vi "Select Fiducial From Set.vi"(8 "error in":errorcluster, 9 "Selection Criteria":enum16{"Single", "Top", "Bottom"}(ring), 10 "Fiducial Centers":refnum<class "Vec3d Class.lvclass">[](array[class])) -> (0 "error out":errorcluster, 2 "Selected Fiducial":refnum<class "Vec3d Class.lvclass">)   [LabVIEW 2011]
uses:
  Vec3d Class/Vec3d Class.lvclass
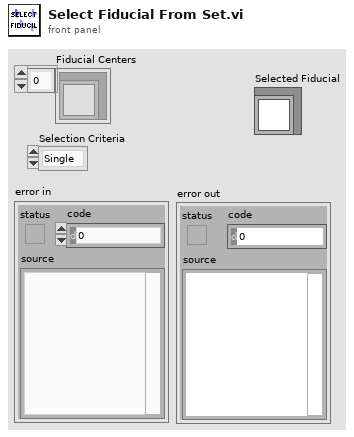
[diagram p1: front panel]
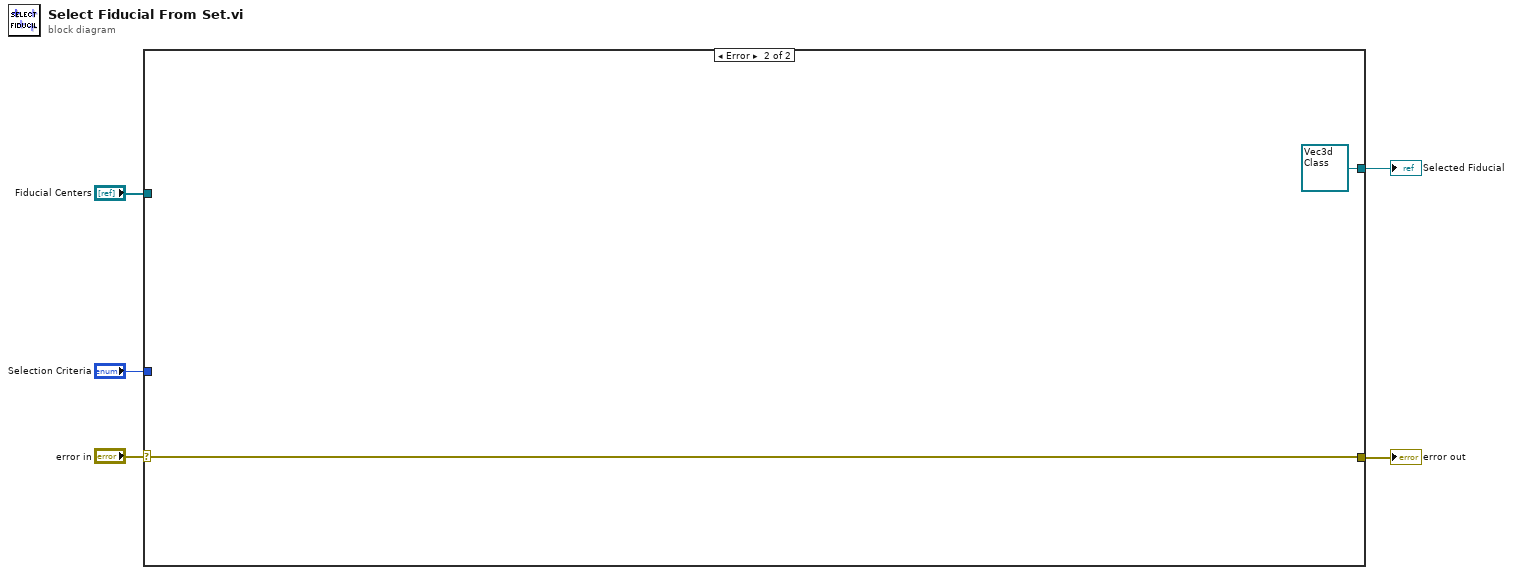
[diagram p0: block diagram]
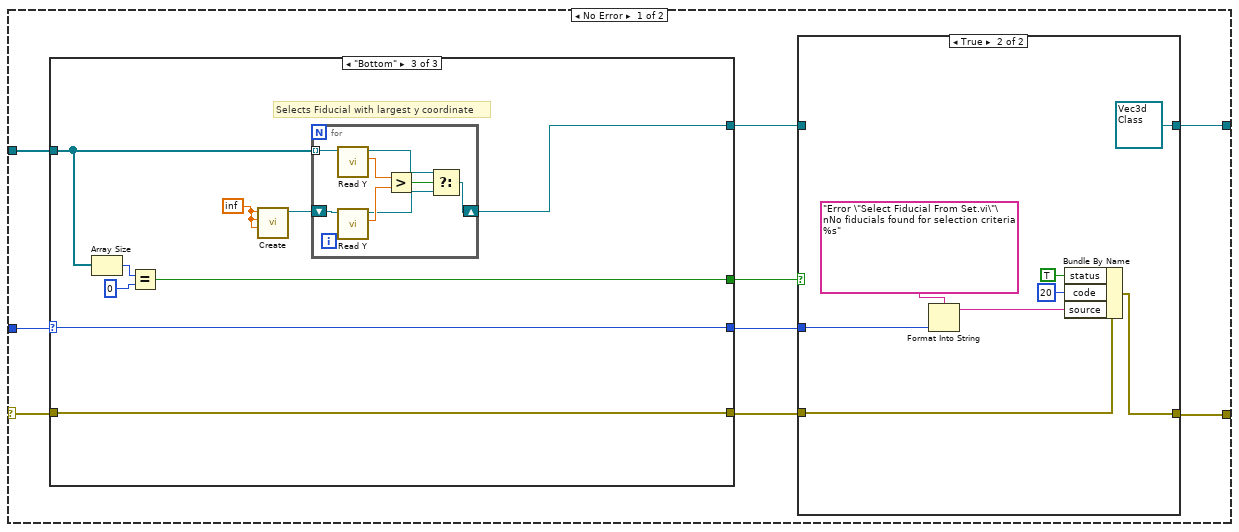
[diagram p2: hidden frame]
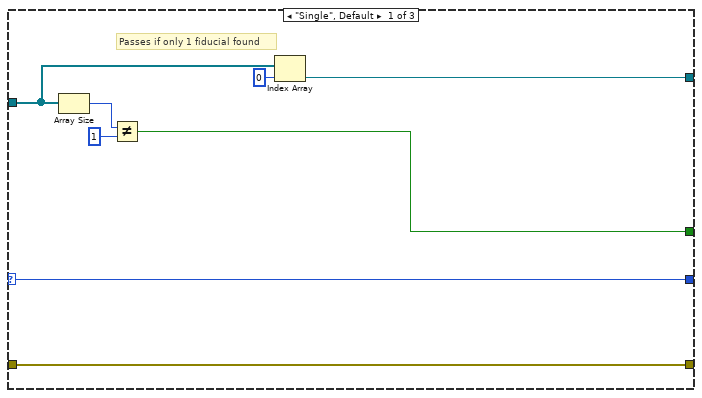
[diagram p3: hidden frame]
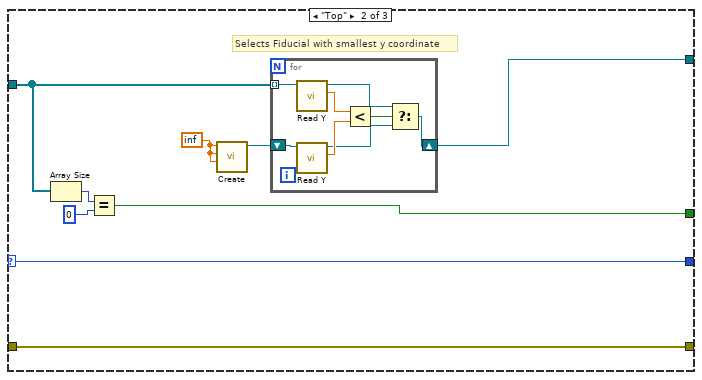
[diagram p4: hidden frame]
diagram:
  n1 = case shown="Error" "error in" {
    selector: "error in" -> [w6 w67]
    tunnel: "Fiducial Centers" -> [w14 _]
    tunnel: [w11 refnum<class "Vec3d Class.lvclass"> refnum ("Vec3d Class out")] -> w4
    tunnel: [w10 w67] -> w3
    tunnel: "Selection Criteria" -> [w7 _]
    frame No Error {
      n2 = case shown="\"Bottom\"" w7 {
        selector: w7 -> [w15 w23 w40]
        tunnel: w14 -> [w20 w30 w47]
        tunnel: w6 -> [w18 w27 w44]
        tunnel: [w19 w31 w48] -> w12
        tunnel: [w18 w27 w44] -> w9
        tunnel: [w16 w24 w41] -> w13
        tunnel: [w15 w23 w40] -> w8
        frame "Single", Default {
          # "Passes if only 1 fiducial found"
          n3 = Array Size(array=w20) -> (size(s)=w21:i32)
          n4 = Not Equal?(x=w21, y=1) -> (x != y?=w16:bool)
          n5 = Index Array(array=w20, index=0) -> (element=w19:refnum<class "Vec3d Class.lvclass">)
        }
        frame "Top" {
          w25 = inf
          # "Selects Fiducial with smallest y coordinate"
          n6 = Array Size(array=w30) -> (size(s)=w28:i32)
          n7 = Equal?(x=w28, y=0) -> (x = y?=w24:bool)
          n8 = call "Create.vi"("Z"=w25, "Y"=w25, "X"=w25) -> ("Vec3d Class out"=w26:refnum<class "Vec3d Class.lvclass">)  [unwired: 7 in, 1 out]
          n9 = for {
            tunnel: w30 -> [w38] mode=indexing
            shift-right: [w32] -> w31
            shift-left: w26 -> [w39]
            n10 = call-dynamic "Read Y.vi"("Vec3d Class in"=w38) -> ("Y"=w37:dbl, "Vec3d Class out"=w34:refnum<class "Vec3d Class.lvclass">)  [unwired: 8 in, 1 out]
            n11 = call-dynamic "Read Y.vi"("Vec3d Class in"=w39) -> ("Y"=w36:dbl, "Vec3d Class out"=w33:refnum<class "Vec3d Class.lvclass">)  [unwired: 8 in, 1 out]
            n12 = Less?(x=w37, y=w36) -> (x < y?=w35:bool)
            n13 = Select(t=w34, s=w35, f=w33) -> (s? t:f=w32:refnum<class "Vec3d Class.lvclass">)
          }
        }
        frame "Bottom" {
          w42 = inf
          # "Selects Fiducial with largest y coordinate"
          n14 = Array Size(array=w47) -> (size(s)=w45:i32)
          n15 = Equal?(x=w45, y=0) -> (x = y?=w41:bool)
          n16 = call "Create.vi"("Z"=w42, "Y"=w42, "X"=w42) -> ("Vec3d Class out"=w43:refnum<class "Vec3d Class.lvclass">)  [unwired: 7 in, 1 out]
          n17 = for {
            tunnel: w47 -> [w55] mode=indexing
            shift-right: [w49] -> w48
            shift-left: w43 -> [w56]
            n18 = call-dynamic "Read Y.vi"("Vec3d Class in"=w55) -> ("Y"=w54:dbl, "Vec3d Class out"=w51:refnum<class "Vec3d Class.lvclass">)  [unwired: 8 in, 1 out]
            n19 = call-dynamic "Read Y.vi"("Vec3d Class in"=w56) -> ("Y"=w53:dbl, "Vec3d Class out"=w50:refnum<class "Vec3d Class.lvclass">)  [unwired: 8 in, 1 out]
            n20 = Greater?(x=w54, y=w53) -> (0:w52:bool)
            n21 = Select(t=w51, s=w52, f=w50) -> (s? t:f=w49:refnum<class "Vec3d Class.lvclass">)
          }
        }
      }
      n22 = case shown="True" w13 {
        tunnel: w12 -> [w57 _]
        tunnel: [w57 refnum<class "Vec3d Class.lvclass"> refnum ("Vec3d Class out")] -> w11
        tunnel: [w58 w60] -> w10
        tunnel: w9 -> [w58 w59]
        tunnel: w8 -> [_ w61]
        frame False {
          # "No Error"
        }
        frame True {
          n23 = Format Into String(format string="Error \"Select Fiducial From Set.vi\"\nNo fiducials found for selection criteria %s" ("source"), w61) -> (resulting string=w62:string)  [unwired: 2 in, 1 out]
          n24 = Bundle By Name(cluster=w59, "status"=TRUE, "code"=20, "source"=w62) -> (w60:errorcluster)
        }
      }
    }
    frame Error {
    }
  }
  "Selected Fiducial" <- w4
  "error out" <- w3
